vi "CMC_ERROR_OUTPUT.vi"() -> ()   [LabVIEW 2013]
panel:
  in  "Frequency":dbl=10.1
  out "Waveform Graph":dynamicdata(graph)
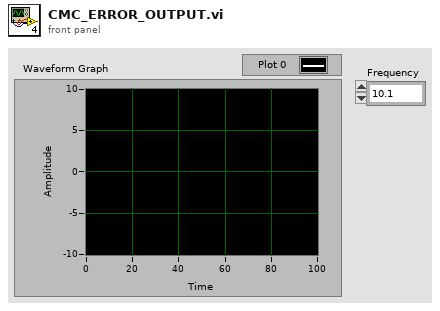
[diagram p1: front panel]
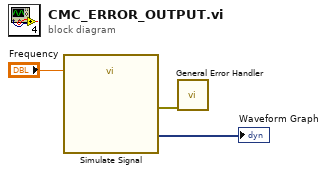
[diagram p0: block diagram]
diagram:
  n1 = call "Simulate Signal"("Frequency"="Frequency") -> ("Sine"=→"Waveform Graph":dynamicdata, "error out"=w1:errorcluster)  [unwired: 13 in]
  n2 = call <vilib>:"General Error Handler.vi"("error in (no error)"=w1) -> ()  [unwired: 10 in, 5 out]
